vi "Read Start.vi"(8 "error in (no error)":errorcluster, 9 "Stream in":refnum<k5>, 11 "Request in":refnum<class "Request.lvclass">) -> (0 "error out":errorcluster, 1 "Stream out":refnum<k5>, 3 "Request out":refnum<class "Request.lvclass">)   [LabVIEW 2020, in "HTTP Utils.lvlib" / "Request.lvclass"]
uses:
  Request.lvclass
  Method.ctl
  Request.lvclass/Request.ctl
  HTTP Utils.lvlib
  lv-uri/URI/URI/URI.lvclass
  lv-uri/URI/URI.lvlib
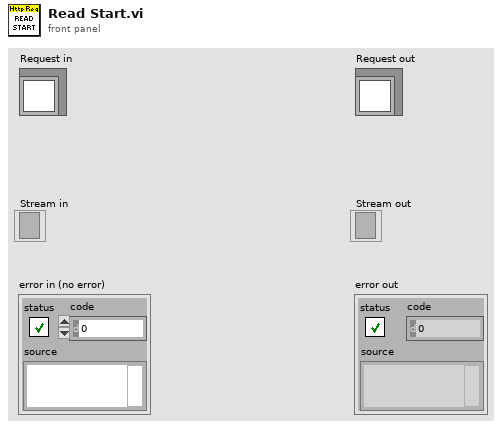
[diagram p1: front panel]
types:
  T1 = typedef "HTTP Utils.lvlib/Method.ctl" = enum16{"GET", "HEAD", "POST", "PUT", "DELETE", "CONNECT", "OPTIONS", "TRACE", "PATCH"}
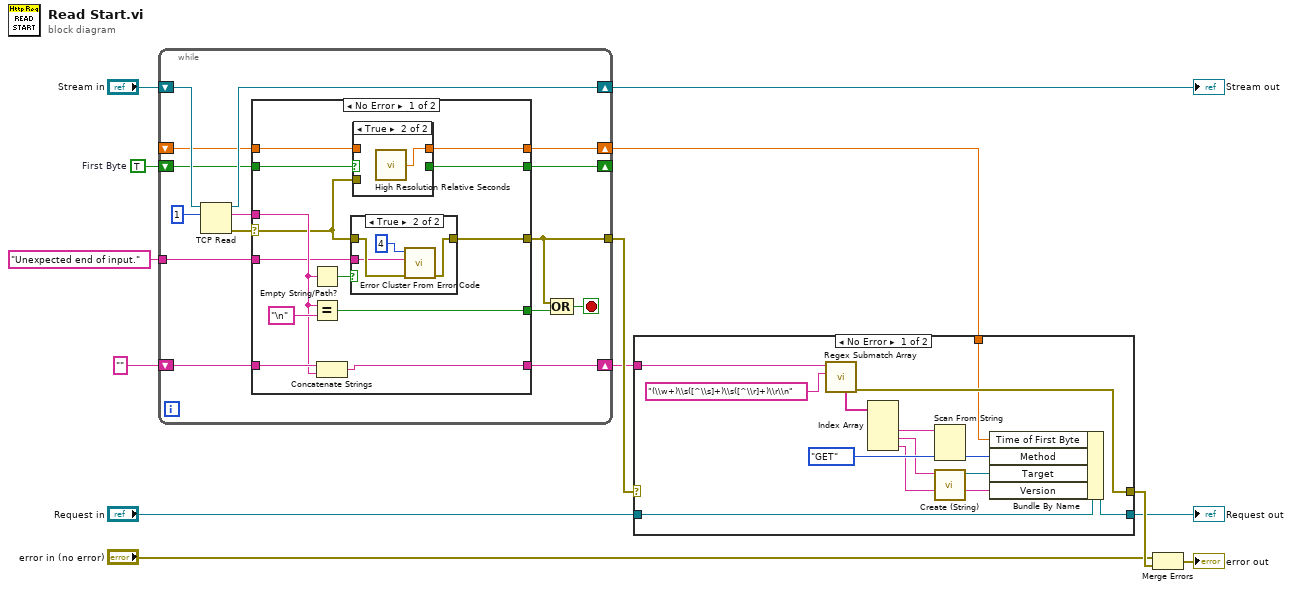
[diagram p0: block diagram]
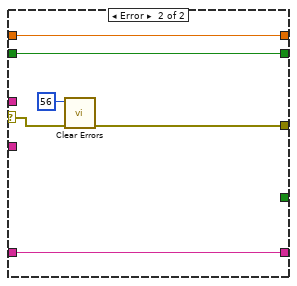
[diagram p4: hidden frame]
diagram:
  w1 = TRUE  # First Byte
  n1 = while {
    shift-right: [w27] -> w11
    shift-left: "Stream in" -> [w28]
    shift-right: [w24] -> w8
    shift-left: "" -> [w26]
    tunnel: [w14] -> w13
    tunnel: "Unexpected end of input." -> [w22]
    shift-right: [w21] -> w2
    shift-left: _ -> [w20]
    shift-right: [w18] -> _
    shift-left: w1 -> [w19]
    stop <- w15 stop-if-true
    n2 = TCP Read(connection ID=w28, bytes to read=1 ("Count")) -> (connection ID out=w27:refnum<k5>, data out=w23:string, error out=w17:errorcluster)  [unwired: 3 in]
    n3 = case shown="No Error" w17 {
      selector: w17 -> [w30 w55]
      tunnel: w26 -> [w40 w50]
      tunnel: [w39 w50] -> w24
      tunnel: w23 -> [w38 _]
      tunnel: [w36 w54] -> w14
      tunnel: w22 -> [w35 _]
      tunnel: [w34 w52] -> w21
      tunnel: w20 -> [w33 w52]
      tunnel: w19 -> [w32 w51]
      tunnel: [w31 w51] -> w18
      tunnel: [w29 _] -> w16
      frame No Error {
        n4 = Empty String/Path?(string/path=w38) -> (empty?=w37:bool)
        n5 = Equal?(x=w38, y="\n") -> (x = y?=w29:bool)
        n6 = Concatenate Strings(w40, w38) -> (w39:string)
        n7 = case shown="True" w37 {
          tunnel: w30 -> [w45 w47]
          tunnel: [w45 w49] -> w36
          tunnel: w35 -> [_ w46]
          frame False {
          }
          frame True {
            n8 = call <vilib>:"Error Cluster From Error Code.vi"("error in (no error)"=w47, "error message (\"\")"=w46, "error code (0)"=4) -> ("error out"=w49:errorcluster)  [unwired: 6 in]
          }
        }
        n9 = case shown="True" w32 {
          selector: w32 -> [w42 _]
          tunnel: w30 -> [_ _]
          tunnel: [w43 w44] -> w34
          tunnel: w33 -> [w43 _]
          tunnel: [w42 _] -> w31
          frame False {
          }
          frame True {
            n10 = call <vilib>:"High Resolution Relative Seconds.vi"() -> ("relative seconds"=w44:dbl)
          }
        }
      }
      frame Error {
        n11 = call <vilib>:"Clear Errors.vi"("error in (no error)"=w55, "specific error code to clear (0: all)"=56) -> ("error out"=w54:errorcluster)  [unwired: 4 in, 1 out]
      }
    }
    n12 = Compound Arithmetic op=OR(w14, w16) -> (w15:bool)
  }
  "Stream out" <- w11
  n13 = case shown="No Error" w13 {
    selector: w13 -> [_ w70]
    tunnel: w8 -> [w62 _]
    tunnel: "Request in" -> [w61 w69]
    tunnel: [w60 w69] -> w4
    tunnel: [w59 w70] -> w7
    tunnel: w2 -> [w58 _]
    frame No Error {
      n14 = call "Regex Submatch Array.vi"("regular expression"="(\\w+)\\s([^\\s]+)\\s([^\\r]+)\\r\\n", "string"=w62) -> ("error out"=w59:errorcluster, "matches"=w65:string[])  [unwired: 5 in, 3 out]
      n15 = Index Array(array=w65) -> (element #2=w64:string, element #3=w57:string, element #4=w63:string)  [unwired: 4 in, 1 out]
      n16 = Scan From String(input string=w64, default 1=Method."GET" ("Method")) -> (output 1=w67:T1)  [unwired: 3 in, 3 out]
      n17 = call "Create (String).vi"("URI String"=w57) -> ("URI out"=w56:refnum<class "URI.lvclass">)  [unwired: 9 in, 1 out]
      n18 = Bundle By Name(cluster=w61, "Time of First Byte"=w58, "Method"=w67, "Target"=w56, "Version"=w63) -> (w60:refnum<class "Request.lvclass">)
    }
    frame Error {
    }
  }
  "Request out" <- w4
  n19 = Merge Errors("error in (no error)", w7) -> (→"error out":errorcluster)
